vi "[FGEN]Set Frequency.vi"() -> (2 "Freq in range?":bool, 3 "Frequency":dbl)   [LabVIEW 2019]
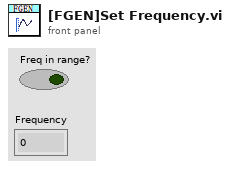
[diagram p1: front panel]
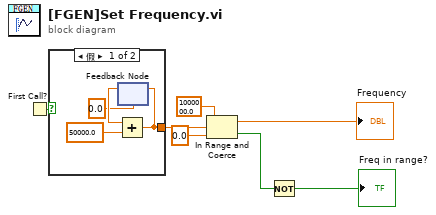
[diagram p0: block diagram]
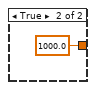
[diagram p2: hidden frame]
diagram:
  n1 = First Call?() -> (First Call?: T/F=w4:bool)
  n2 = case shown="假" w4 {
    tunnel: [w8 1000.0] -> w5
    frame False {
      n3 = feedback #1(0.0) -> (w10:dbl)
      n4 = Add(x=w10, y=50000.0) -> (x+y=w8:dbl)
      n5 = feedback-in #1(w8) -> ()
    }
    frame True {
    }
  }
  n6 = In Range and Coerce(upper limit=1000000.0, x=w5, lower limit=0.0) -> (coerced(x)=→"Frequency":dbl, In Range?=w2:bool)
  n7 = Not(x=w2) -> (.not. x?=→"Freq in range?":bool)
